vi "Fetch (Measurements).vi"(0 "VISA resource name":refnum<visa-resource-name>, 5 "Timeout (10000 ms)":i32=10000 format="%#.6g", 11 "error in (no error)":errorcluster) -> (3 "Voltage":sgl[](array[numeric]), 4 "VISA resource name out":refnum<visa-resource-name>, 6 "Current":sgl[](array[numeric]), 8 "Resistance":sgl[](array[numeric]), 10 "Timestamp":sgl[](array[numeric]), 14 "Status":sgl[](array[numeric]), 15 "error out":errorcluster)   [LabVIEW 2014, in "Keithley 24XX.lvlib"]
doc: "Fetches data for voltage, current, resistance, timestamp, and status. These readings are then provided in separate arrays for each type of reading.\n\n<B>Note</B> Use this VI only with other low-level VIs. The high-level VIs automatically incorporate this functionality. This VI does not check the instrument status. If you want to check the instrument status, call the Error Query VI at the conclusion of the sequence."
uses:
  Keithley 24XX.lvlib
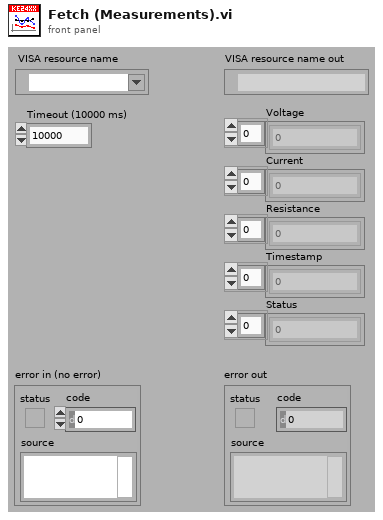
[diagram p1: front panel]
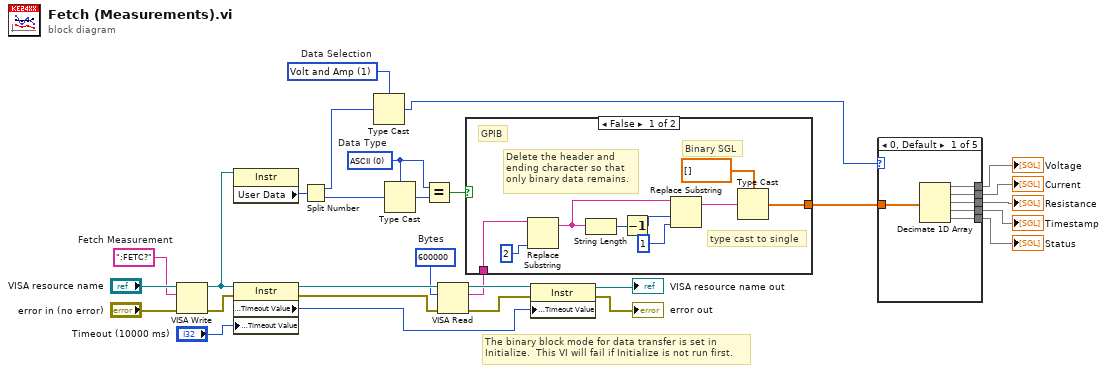
[diagram p0: block diagram]
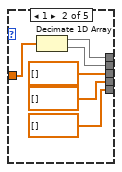
[diagram p2: hidden frame]
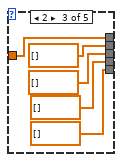
[diagram p3: hidden frame]
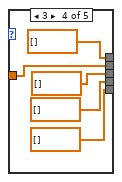
[diagram p4: hidden frame]
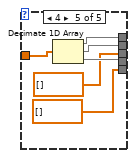
[diagram p5: hidden frame]
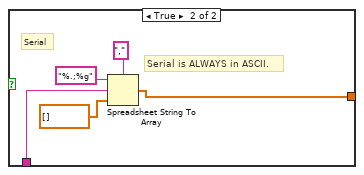
[diagram p6: hidden frame]
diagram:
  w8 = u16 1 items=["All", "Volt and Amp", "Volt", "Amp"]  # Data Selection
  w11 = u16 0 items=["ASCII", "Binary (Single Precision Real)"]  # Data Type
  w27 = ":FETC?"  # Fetch Measurement
  w17 = u32 600000  # Bytes
  # "The binary block mode for data transfer is set in Initialize.  This VI will fail if Initialize is not run first."
  n1 = VISA Write(VISA resource name="VISA resource name", write buffer=w27, error in (no error)="error in (no error)") -> (VISA resource name out=w10:refnum<visa-resource-name>, error out=w26:errorcluster)  [unwired: 1 out]
  n2 = property class="Instr"(reference=w10) -> ("User Data"=w14:u32)  [unwired: 2 in, 1 out]
  n3 = property class="Instr"(reference=w10, error in=w26, "General Settings:Timeout Value"="Timeout (10000 ms)") -> (reference out=w25:refnum<visa-resource-name>, error out=w24:errorcluster, "General Settings:Timeout Value"=w20:u32)
  n4 = Split Number(x=w14) -> (hi(x)=w9:u16, lo(x)=w13:u16)
  n5 = Type Cast(type=w8, x=w9) -> (*(type *) &x=w6:u16)
  n6 = Type Cast(type=w11, x=w13) -> (*(type *) &x=w12:u16)
  n7 = Equal?(x=w11, y=w12) -> (x = y?=w7:bool)
  n8 = VISA Read(VISA resource name=w25, byte count=w17, error in (no error)=w24) -> (VISA resource name out=w22:refnum<visa-resource-name>, read buffer=w16:string, error out=w21:errorcluster)  [unwired: 1 out]
  n9 = case shown="False" w7 {
    tunnel: w16 -> [w38 w43]
    tunnel: [w30 w39] -> w15
    frame False {
      # "Binary SGL"
      # "Delete the header and ending character so that only binary data remains."
      # "GPIB"
      # "type cast to single"
      n10 = Replace Substring(2:2 ("length (len. of substring)"), 5:w38) -> (1:w36:string)  [unwired: 2 in, 1 out]
      n11 = String Length(string=w36) -> (length=w35:i32)
      n12 = Decrement(x=w35) -> (x-1=w34:i32)
      n13 = Replace Substring(2:1 ("length (len. of substring)"), 3:w34, 5:w36) -> (1:w32:string)  [unwired: 1 in, 1 out]
      n14 = Type Cast(type=sgl[] [], x=w32) -> (*(type *) &x=w30:sgl[])
    }
    frame True {
      # "Serial is ALWAYS in ASCII."
      # "Serial"
      n15 = Spreadsheet String To Array(delimiter (Tab)=",", format string="%.;%g", spreadsheet string=w43, array type (2D Dbl)=sgl[] []) -> (array=w39:sgl[])
    }
  }
  n16 = property class="Instr"(reference=w22, error in=w21, "General Settings:Timeout Value"=w20) -> (reference out=→"VISA resource name out":refnum<visa-resource-name>, error out=→"error out":errorcluster)
  n17 = case shown="0, Default" w6 {
    tunnel: w15 -> [w49 w55 w60 w65 w71]
    tunnel: [w48 w54 w60 sgl[] [] w70] -> w5
    tunnel: [w47 w53 sgl[] [] w65 w69] -> w4
    tunnel: [w46 sgl[] [] sgl[] [] sgl[] [] sgl[] []] -> w3
    tunnel: [w45 sgl[] [] sgl[] [] sgl[] [] w68] -> w2
    tunnel: [w44 sgl[] [] sgl[] [] sgl[] [] sgl[] []] -> w1
    frame 0, Default {
      n18 = Decimate 1D Array(w49) -> (w48:sgl[], w47:sgl[], w46:sgl[], w45:sgl[], w44:sgl[])
    }
    frame 1 {
      n19 = Decimate 1D Array(w55) -> (w54:sgl[], w53:sgl[])
    }
    frame 2 {
    }
    frame 3 {
    }
    frame 4 {
      n20 = Decimate 1D Array(w71) -> (w70:sgl[], w69:sgl[], w68:sgl[])
    }
  }
  "Voltage" <- w5
  "Current" <- w4
  "Resistance" <- w3
  "Timestamp" <- w2
  "Status" <- w1
